vi "write_u8 array.vi"(8 "error in (no error)":errorcluster caption="에러 입력(에러 없음)", 9 "data to write":u8[](array[numeric]), 10 "start address":u32, 11 "I2C 입력":refnum<class "I2C.lvclass">) -> (0 "error out":errorcluster caption="에러 출력", 1 "data out":u8[](array[numeric]), 2 "log_multiple line":string[](array[string]), 3 "I2C 출력":refnum<class "I2C.lvclass">, 4 "log_single line":string[](array[string]))   [LabVIEW 2020, in "I2C.lvclass"]
uses:
  I2C.lvclass
  I2C.lvclass/I2C.ctl
  SubVIs/Serial/Controls/(Ctrl)Serial_Write Read Option.ctl
  Controls/(Ctrl)log & script_rw enum.ctl
  Accessors/Read address byte.vi
  Accessors/Read clock rate.vi
  Accessors/Read slave address.vi
  Variables/(Var)System Variables.vi
  SubVIs/Serial/Instance VIs/(SubVI)Serial_Write-Read.vi
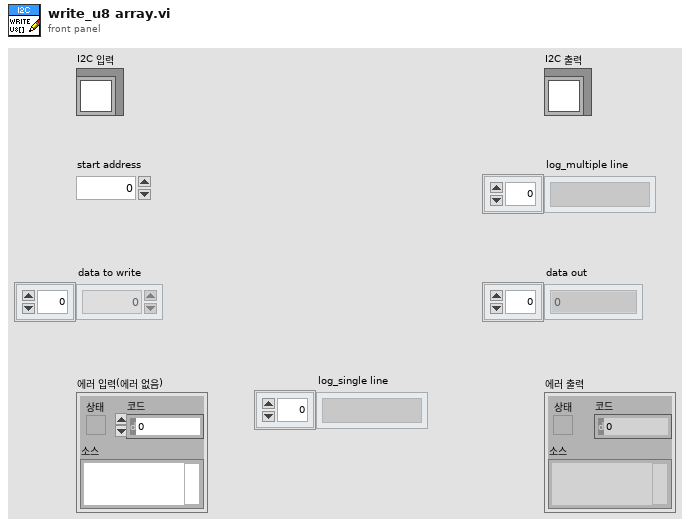
[diagram p1: front panel]
types:
  T1 = typedef "I2C.lvclass/(Ctrl)log & script_rw enum.ctl" = enum16{"Read", "Write"}
  T2 = typedef "(Ctrl)Serial_Write Read Option.ctl" = cluster{"Echo Request":bool, "Header Verification":bool, "Checksum Verification":bool, "User Code Verifiaction":bool}
  T3 = typedef "IC I2C Clock Rate.ctl" = enum8{"50khz", "100khz", "400khz", "1Mhz", "1.2Mhz"}
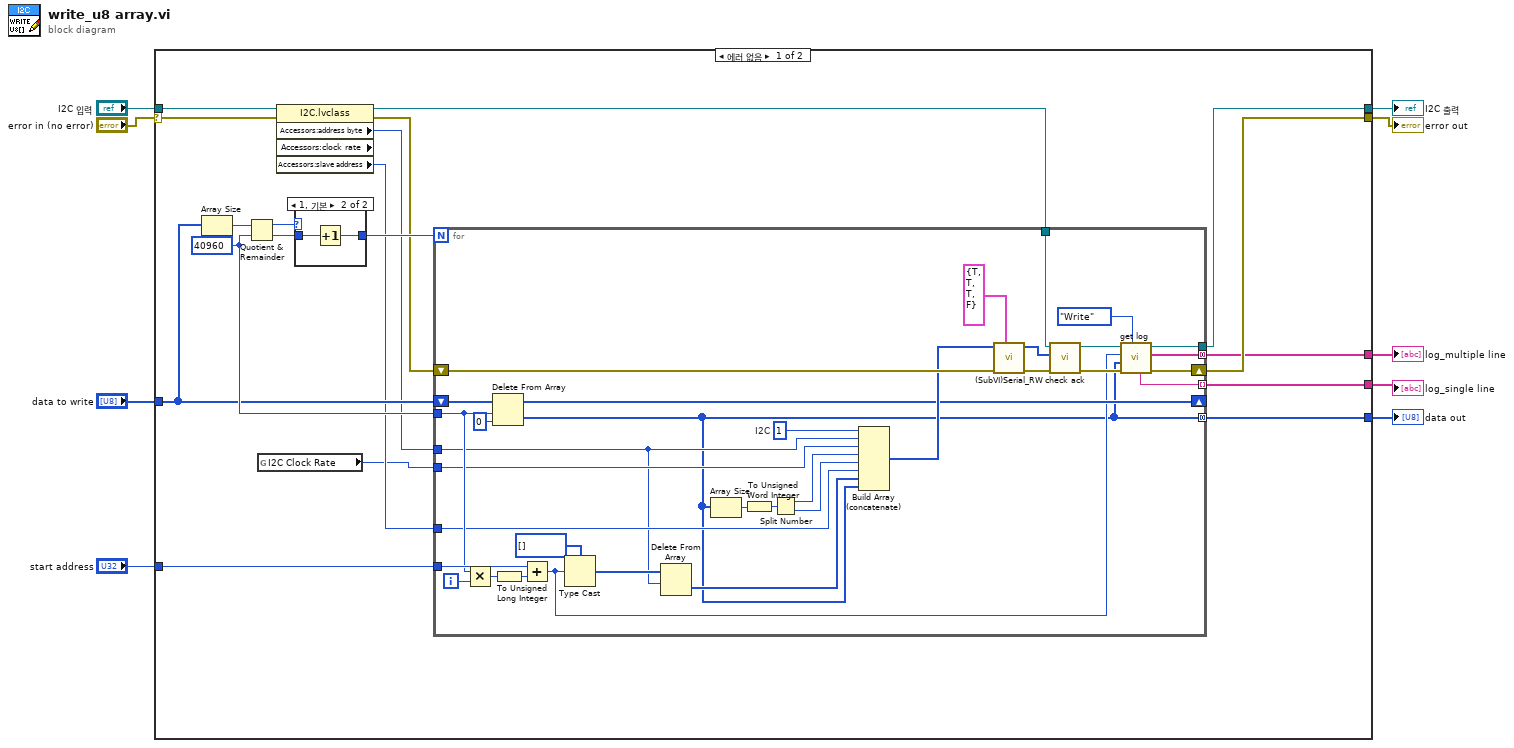
[diagram p0: block diagram]
diagram:
  n1 = case shown="에러 없음" "error in (no error)" {
    selector: "error in (no error)" -> [w27 w67]
    tunnel: [w18 w67] -> w8
    tunnel: [w13 w66] -> w6
    tunnel: "I2C 입력" -> [w28 w66]
    tunnel: "data to write" -> [w21 _]
    tunnel: "start address" -> [w20 _]
    tunnel: [w15 _] -> w3
    tunnel: [w12 _] -> w2
    tunnel: [w11 _] -> w1
    frame No Error {
      w22 = 40960 ("y")
      n2 = Array Size(array=w21) -> (size(s)=w23:i32)
      n3 = Quotient & Remainder(x=w23, y=w22) -> (x-y*floor(x/y)=w24:i32, floor(x/y)=w25:i32)
      n4 = global read "(Var)System Variables.vi" "I2C Clock Rate"() -> (w10:T3)
      n5 = property class="I2C.lvclass" props=["Accessors:address byte", "Accessors:clock rate", "Accessors:slave address"](reference=w28, error in=w27) -> (reference out=w14:refnum<class "I2C.lvclass">, error out=w19:errorcluster, "Accessors:address byte"=w16:u8, "Accessors:slave address"=w17:u8)  [unwired: 1 out]
      n6 = case shown="1, 기본" w24 {
        tunnel: w25 -> [w63 w65]
        tunnel: [w63 w64] -> w26
        frame 0 {
        }
        frame 1, Default {
          n7 = Increment(x=w65) -> (x+1=w64:i32)
        }
      }
      n8 = for {
        N: w26 -> [_]
        tunnel: w20 -> [w46]
        shift-right: [w36] -> w18
        shift-left: w19 -> [w62]
        shift-right: [w49] -> _
        shift-left: w21 -> [w51]
        tunnel: w22 -> [w44]
        tunnel: [w31] -> w15 mode=concatenating
        tunnel: w17 -> [w43]
        tunnel: w10 -> [w40]
        tunnel: w16 -> [w37]
        tunnel: w14 -> [w39]
        tunnel: [w34] -> w13
        tunnel: [w30] -> w12 mode=concatenating
        tunnel: [w29] -> w11 mode=indexing
        i -> [w45]
        w60 = u8 1  # I2C
        n9 = Multiply(x=w44, y=w45) -> (x*y=w48:i32)
        n10 = Delete From Array(array=w51, length=w44, index=0 ("인덱스")) -> (deleted portion=w31:u8[], array with subset deleted=w49:u8[])
        n11 = To Unsigned Long Integer(number=w48) -> (unsigned 32bit integer=w47:u32)
        n12 = Add(x=w46, y=w47) -> (x+y=w32:u32)
        n13 = Type Cast(type=u8[] [] ("타입"), x=w32) -> (*(type *) &x=w38:u8[])
        n14 = Delete From Array(array=w38, length=w37) -> (deleted portion=w41:u8[])  [unwired: 1 in, 1 out]
        n15 = Array Size(array=w31) -> (size(s)=w61:i32)
        n16 = To Unsigned Word Integer(number=w61) -> (unsigned 16bit integer=w57:u16)
        n17 = Split Number(x=w57) -> (hi(x)=w59:u8, lo(x)=w58:u8)
        n18 = Build Array (concatenate)(w60, w37, w40, w59, w58, w43, w41, w31) -> (w52:u8[])
        n19 = call-poly "(SubVI)Serial_RW.vi"("Option"=T2 {"Echo Request"=TRUE, "Header Verification"=TRUE, "Checksum Verification"=TRUE, "User Code Verifiaction"=FALSE}, "error in (no error)"=w62, "Data to Write"=w52) -> ("error out"=w55:errorcluster, "Read Data"=w54:u8[])  [unwired: 6 in, 1 out]
        n20 = call-dynamic "check ack.vi"("error in (no error)"=w55, "Read Data"=w54, "I2C 입력"=w39) -> ("error out"=w56:errorcluster, "I2C 출력"=w35:refnum<class "I2C.lvclass">)  [unwired: 6 in, 1 out]
        n21 = call-dynamic "get log.vi"("rw"=(Ctrl)log_&_script_rw_enum."Write", "error in (no error)"=w56, "data"=w31, "start addr"=w32, "I2C 입력"=w35) -> ("error out"=w36:errorcluster, "log_multiple line"=w30:string[], "I2C 출력"=w34:refnum<class "I2C.lvclass">, "log_single line"=w29:string)  [unwired: 3 in]
      }
    }
    frame Error {
    }
  }
  "error out" <- w8
  "I2C 출력" <- w6
  "data out" <- w3
  "log_multiple line" <- w2
  "log_single line" <- w1
